vi "String - Extract Mid String.vi"(0 "String":string, 7 "Start search string":string, 11 "End search string":string, 12 "Offset":i32) -> (3 "Start String Found":bool, 4 "String - Before":string, 6 "String - Start":string, 8 "String - Middle":string, 10 "String - End":string, 14 "End String Found":bool, 15 "String - After":string)   [LabVIEW 2011]
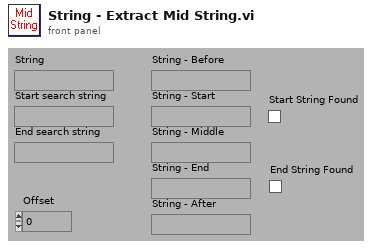
[diagram p1: front panel]
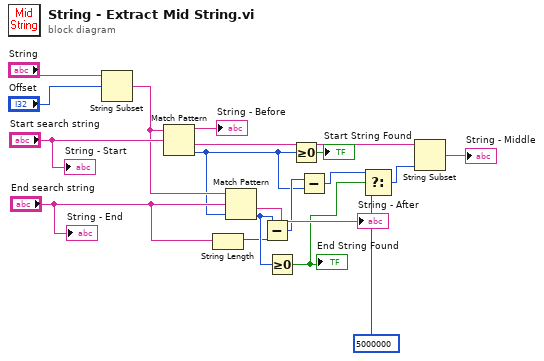
[diagram p0: block diagram]
diagram:
  n1 = String Subset(string="String", offset (0)="Offset") -> (substring=w11:string)  [unwired: 1 in]
  n2 = Match Pattern(string=w11, regular expression="Start search string") -> (before substring=→"String - Before":string, after substring=w16:string, offset past match=w8:i32)  [unwired: 1 in, 1 out]
  n3 = String Length(string="End search string") -> (length=w2:i32)
  n4 = Match Pattern(string=w11, regular expression="End search string", offset (0)=w8) -> (after substring=→"String - After":string, offset past match=w6:i32)  [unwired: 2 out]
  n5 = Subtract(x=w6, y=w2) -> (x-y=w9:i32)
  n6 = Greater Or Equal To 0?(x=w6) -> (x >= 0?=w5:bool)
  "End String Found" <- w5
  n7 = Greater Or Equal To 0?(x=w8) -> (x >= 0?=→"Start String Found":bool)
  n8 = Subtract(x=w9, y=w8) -> (x-y=w4:i32)
  n9 = Select(t=w4, s=w5, f=5000000) -> (s? t:f=w3:i32)
  n10 = String Subset(string=w16, length (rest)=w3) -> (substring=→"String - Middle":string)  [unwired: 1 in]
  "String - Start" <- "Start search string"
  "String - End" <- "End search string"
